vi "drive_begin.vi"   [LabVIEW 2013]
uses:
  <vilib>/Rock Robotics/WPI/CAN/Jaguar/SubVIs/WPI_CANJaguar_ControlMode.ctl
  <vilib>/Rock Robotics/WPI/MotorControl/WPI_MotorControlOpenCANJaguar.vi
types:
  T1 = typedef "WPI_CANJaguar_ControlMode.ctl" = enum8{"Percent VBus", "Current", "Speed", "Position", "Voltage"}
  T2 = typedef "WPI_MotorControlDeviceRef.ctl" = cluster{"DeviceStatus":errorcluster, "Type":enum16{"PWM", "CAN"}, "PWM":cluster{"Digital Module":T3, "PWM Channel":T4, "DeadBand":T5}, "CAN":cluster{"Device Number":u8, "Control Mode":T1, "Semaphore":T6, "Max Vout":dbl}, "Invert":bool, "TransformRef":T7, "InvTransformRef":T7}
  T3 = typedef "FPGA_TypedefDigitalModule.ctl" = enum16{"Digital Module 1", "Digital Module 2"}
  T4 = typedef "FPGA_DIOPWMChannel.ctl" = enum8{"PWM 1", "PWM 2", "PWM 3", "PWM 4", "PWM 5", "PWM 6", "PWM 7", "PWM 8", "PWM 9", "PWM 10", "Invalid"}
  T5 = typedef "WPI_PWMDeadband.ctl" = cluster{"Name":string, "maxPositivePwm":i32, "minPositivePwm":i32, "centerPwm":i32, "maxNegativePwm":i32, "minNegativePwm":i32, "angularRange":u16}
  T6 = typedef "Semaphore RefNum" = refnum<k1>
  T7 = typedef "WPI_PWMTransform_ConPane.ctl" = refnum<vi>
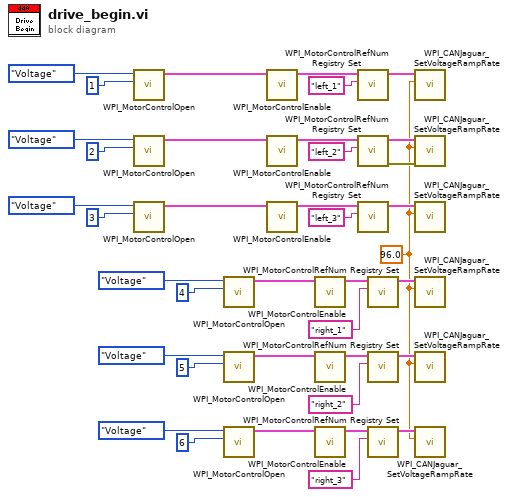
[diagram p0: block diagram]
diagram:
  w1 = 96.0 ("VoltageRampRate (V/s)")
  n1 = call-poly <vilib>:"WPI_MotorControlOpen.vi"("Device Number"=u8 1, "Control Mode"=WPI_CANJaguar_ControlMode."Voltage") -> ("MotorControlDeviceRef"=w38:T2)  [unwired: 8 in, 1 out]
  n2 = call-poly <vilib>:"WPI_MotorControlOpen.vi"("Device Number"=u8 2, "Control Mode"=WPI_CANJaguar_ControlMode."Voltage") -> ("MotorControlDeviceRef"=w28:T2)  [unwired: 8 in, 1 out]
  n3 = call-poly <vilib>:"WPI_MotorControlOpen.vi"("Device Number"=u8 3, "Control Mode"=WPI_CANJaguar_ControlMode."Voltage") -> ("MotorControlDeviceRef"=w33:T2)  [unwired: 8 in, 1 out]
  n4 = call-poly <vilib>:"WPI_MotorControlOpen.vi"("Device Number"=u8 4, "Control Mode"=WPI_CANJaguar_ControlMode."Voltage") -> ("MotorControlDeviceRef"=w23:T2)  [unwired: 8 in, 1 out]
  n5 = call-poly <vilib>:"WPI_MotorControlOpen.vi"("Device Number"=u8 5, "Control Mode"=WPI_CANJaguar_ControlMode."Voltage") -> ("MotorControlDeviceRef"=w13:T2)  [unwired: 8 in, 1 out]
  n6 = call-poly <vilib>:"WPI_MotorControlOpen.vi"("Device Number"=u8 6, "Control Mode"=WPI_CANJaguar_ControlMode."Voltage") -> ("MotorControlDeviceRef"=w18:T2)  [unwired: 8 in, 1 out]
  n7 = call <vilib>:"WPI_MotorControlEnable.vi"("CAN Jaguar Ref"=w38) -> ("CAN Jaguar Ref Out"=w37:T2)  [unwired: 9 in, 1 out]
  n8 = call <vilib>:"WPI_MotorControlEnable.vi"("CAN Jaguar Ref"=w28) -> ("CAN Jaguar Ref Out"=w27:T2)  [unwired: 9 in, 1 out]
  n9 = call <vilib>:"WPI_MotorControlEnable.vi"("CAN Jaguar Ref"=w33) -> ("CAN Jaguar Ref Out"=w32:T2)  [unwired: 9 in, 1 out]
  n10 = call <vilib>:"WPI_MotorControlEnable.vi"("CAN Jaguar Ref"=w23) -> ("CAN Jaguar Ref Out"=w22:T2)  [unwired: 9 in, 1 out]
  n11 = call <vilib>:"WPI_MotorControlEnable.vi"("CAN Jaguar Ref"=w13) -> ("CAN Jaguar Ref Out"=w12:T2)  [unwired: 9 in, 1 out]
  n12 = call <vilib>:"WPI_MotorControlEnable.vi"("CAN Jaguar Ref"=w18) -> ("CAN Jaguar Ref Out"=w17:T2)  [unwired: 9 in, 1 out]
  n13 = call <vilib>:"WPI_MotorControlRefNum Registry Set.vi"("refnum name"="left_1", "MotorControlDevRef"=w37) -> ("MotorControlDevRef"=w2:T2)  [unwired: 8 in, 1 out]
  n14 = call <vilib>:"WPI_MotorControlRefNum Registry Set.vi"("refnum name"="left_2", "MotorControlDevRef"=w27) -> ("error out"=w8:errorcluster, "MotorControlDevRef"=w7:T2)  [unwired: 8 in]
  n15 = call <vilib>:"WPI_MotorControlRefNum Registry Set.vi"("refnum name"="left_3", "MotorControlDevRef"=w32) -> ("MotorControlDevRef"=w3:T2)  [unwired: 8 in, 1 out]
  n16 = call <vilib>:"WPI_MotorControlRefNum Registry Set.vi"("refnum name"="right_1", "MotorControlDevRef"=w22) -> ("MotorControlDevRef"=w4:T2)  [unwired: 8 in, 1 out]
  n17 = call <vilib>:"WPI_MotorControlRefNum Registry Set.vi"("refnum name"="right_2", "MotorControlDevRef"=w12) -> ("MotorControlDevRef"=w5:T2)  [unwired: 8 in, 1 out]
  n18 = call <vilib>:"WPI_MotorControlRefNum Registry Set.vi"("refnum name"="right_3", "MotorControlDevRef"=w17) -> ("MotorControlDevRef"=w6:T2)  [unwired: 8 in, 1 out]
  n19 = call <vilib>:"WPI_CANJaguar_SetVoltageRampRate.vi"("VoltageRampRate (V/s)"=w1, "CAN Jaguar Ref"=w2) -> ()  [unwired: 8 in, 2 out]
  n20 = call <vilib>:"WPI_CANJaguar_SetVoltageRampRate.vi"("error in (no error)"=w8, "VoltageRampRate (V/s)"=w1, "CAN Jaguar Ref"=w7) -> ()  [unwired: 7 in, 2 out]
  n21 = call <vilib>:"WPI_CANJaguar_SetVoltageRampRate.vi"("VoltageRampRate (V/s)"=w1, "CAN Jaguar Ref"=w3) -> ()  [unwired: 8 in, 2 out]
  n22 = call <vilib>:"WPI_CANJaguar_SetVoltageRampRate.vi"("VoltageRampRate (V/s)"=w1, "CAN Jaguar Ref"=w4) -> ()  [unwired: 8 in, 2 out]
  n23 = call <vilib>:"WPI_CANJaguar_SetVoltageRampRate.vi"("VoltageRampRate (V/s)"=w1, "CAN Jaguar Ref"=w5) -> ()  [unwired: 8 in, 2 out]
  n24 = call <vilib>:"WPI_CANJaguar_SetVoltageRampRate.vi"("VoltageRampRate (V/s)"=w1, "CAN Jaguar Ref"=w6) -> ()  [unwired: 8 in, 2 out]
